vi "Read Fiducial Definitions.vi"(8 "error in":errorcluster, 10 "Fiducial Type":string, 11 "Config Manager in":refnum<class "Config Manager Class.lvclass">) -> (0 "error out":errorcluster, 2 "Feature Definitions":T1(array[cluster]), 3 "Config Manager out":refnum<class "Config Manager Class.lvclass">)   [LabVIEW 2017, in "Config Manager Class.lvclass"]
uses:
  Config Manager Class.lvclass
  Vec3d Class/Vec3d Class.lvclass
  Config Manager Class.lvclass/Config Manager Class.ctl
  <vilib>/Utility/config.llb/Read Key (String).vi
  <vilib>/Utility/config.llb/NI_LVConfig.lvlib
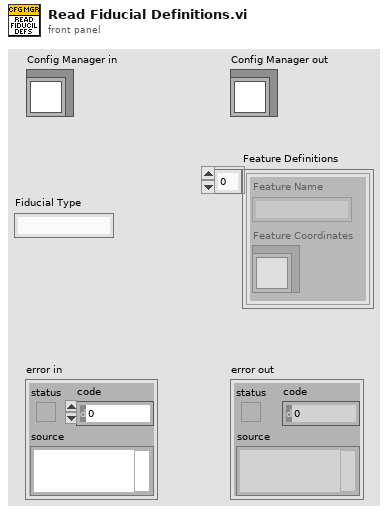
[diagram p1: front panel]
types:
  T1 = cluster{"Feature Coordinates":refnum<class "Vec3d Class.lvclass">, "Feature Name":string}[]
  T2 = cluster{"Feature Coordinates":refnum<class "Vec3d Class.lvclass">, "Feature Name":string}
  T3 = typedef "NI_LVConfig.lvlib/Config Data RefNum.ctl" = refnum<k1>
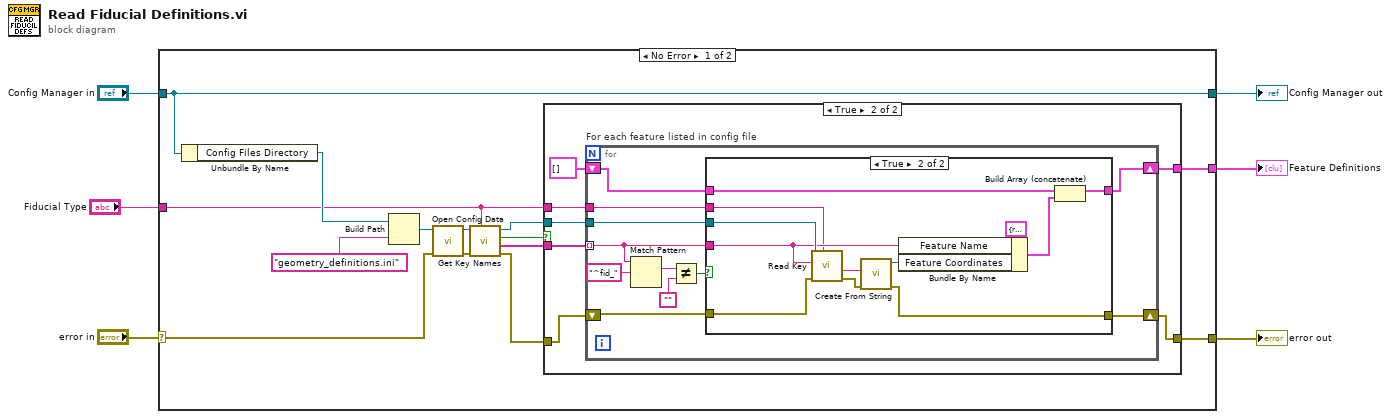
[diagram p0: block diagram]
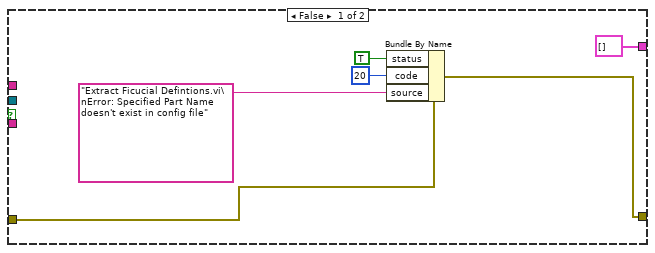
[diagram p2: hidden frame]
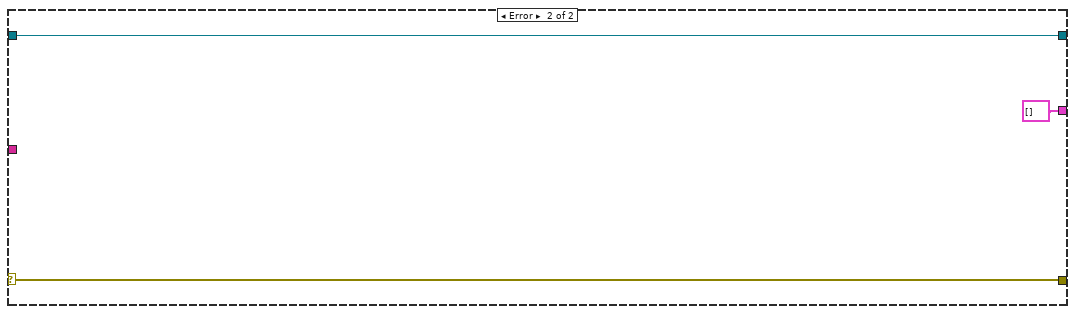
[diagram p4: hidden frame]
diagram:
  n1 = case shown="No Error" "error in" {
    selector: "error in" -> [w10 w61]
    tunnel: [w14 w61] -> w4
    tunnel: [w11 T1 []] -> w6
    tunnel: "Config Manager in" -> [w8 w59]
    tunnel: [w8 w59] -> w2
    tunnel: "Fiducial Type" -> [w7 _]
    frame No Error {
      n2 = Unbundle By Name(w8) -> ("Config Files Directory"=w9:path)
      n3 = Build Path(base path=w9, name or relative path="geometry_definitions.ini") -> (appended path=w19:path)
      n4 = call <vilib>:"Open Config Data.vi"("error in (no error)"=w10, "configuration file path"=w19) -> ("error out"=w17:errorcluster, "refnum"=w18:T3)  [unwired: 7 in, 1 out]
      n5 = call <vilib>:"Get Key Names.vi"("section"=w7, "error in (no error)"=w17, "refnum"=w18) -> ("error out"=w15:errorcluster, "key names"=w13:string[], "section exists?"=w16:bool, "refnum out"=w12:T3)  [unwired: 5 in]
      n6 = case shown="True" w16 {
        tunnel: w15 -> [w22 w31]
        tunnel: [w21 w30] -> w14
        tunnel: w13 -> [_ w32]
        tunnel: w12 -> [_ w33]
        tunnel: [T1 [] w29] -> w11
        tunnel: w7 -> [_ w27]
        frame False {
          n7 = Bundle By Name(cluster=w22, "status"=TRUE, "code"=20, "source"="Extract Ficucial Defintions.vi\nError: Specified Part Name doesn't exist in config file") -> (w21:errorcluster)
        }
        frame True {
          n8 = for "For each feature listed in config file" {
            tunnel: w33 -> [w44]
            tunnel: w32 -> [w41] mode=indexing
            shift-right: [w42] -> w30
            shift-left: w31 -> [w43]
            shift-right: [w35] -> w29
            shift-left: T1 [] -> [w36]
            tunnel: w27 -> [w34]
            n9 = Match Pattern(string=w41, regular expression="^fid_") -> (match substring=w39:string)  [unwired: 1 in, 3 out]
            n10 = Not Equal?(x=w39, y="") -> (x != y?=w37:bool)
            n11 = case shown="True" w37 {
              tunnel: w44 -> [_ w58]
              tunnel: w43 -> [w45 w55]
              tunnel: [w45 w52] -> w42
              tunnel: w41 -> [_ w51]
              tunnel: w36 -> [w46 w50]
              tunnel: [w46 w48] -> w35
              tunnel: w34 -> [_ w47]
              frame False {
              }
              frame True {
                n12 = call-poly <vilib>:"Read Key.vi"("section"=w47, "error in (no error)"=w55, "key"=w51, "refnum"=w58) -> ("error out"=w56:errorcluster, "value"=w57:string)  [unwired: 4 in, 2 out]
                n13 = call "Create From String.vi"("error in"=w56, "Input String"=w57) -> ("error out"=w52:errorcluster, "Vec3d out"=w53:refnum<class "Vec3d Class.lvclass">)  [unwired: 8 in]
                n14 = Bundle By Name(cluster=T2 {"Feature Coordinates"=refnum, "Feature Name"=""} ("Feature Description"), "Feature Name"=w51, "Feature Coordinates"=w53) -> (w49:T2)
                n15 = Build Array (concatenate)(w50, w49) -> (w48:T1)
              }
            }
          }
        }
      }
    }
    frame Error {
    }
  }
  "error out" <- w4
  "Config Manager out" <- w2
  "Feature Definitions" <- w6
